vi "Borda_1.vi"(5 "Entrada":bool) -> (2 "Boolean":bool)   [LabVIEW 2018]
panel:
  in  "Aux Muda":bool
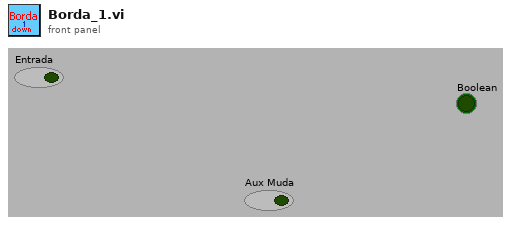
[diagram p1: front panel]
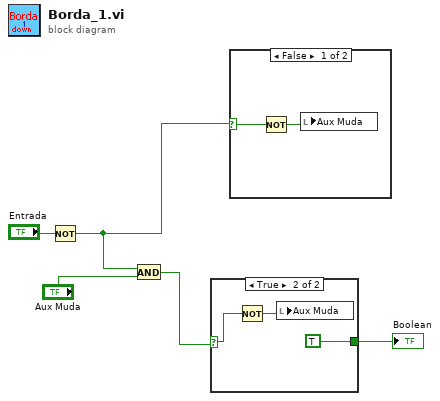
[diagram p0: block diagram]
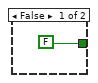
[diagram p3: hidden frame]
diagram:
  n1 = Not(x="Entrada") -> (.not. x?=w1:bool)
  n2 = And(x=w1, y="Aux Muda") -> (x .and. y?=w2:bool)
  n3 = case shown="True" w2 {
    selector: w2 -> [_ w7]
    tunnel: [FALSE ("Boolean") TRUE ("Boolean")] -> w5
    frame False {
    }
    frame True {
      n4 = Not(x=w7) -> (.not. x?=w8:bool)
      n5 = local write "Aux Muda"(w8) -> ()
    }
  }
  "Boolean" <- w5
  n6 = case shown="False" w1 {
    selector: w1 -> [w11 _]
    frame False {
      n7 = Not(x=w11) -> (.not. x?=w10:bool)
      n8 = local write "Aux Muda"(w10) -> ()
    }
    frame True {
    }
  }
